vi "4.vi"() -> ()   [LabVIEW 2018]
panel:
  out "W":dbl
  in  "Z":dbl
  in  "Y":dbl
  in  "X":dbl
  # "some debugging tools :\ncontext help \nprobe \nexecution highlight\nsingle stepping \nbreak points \nretian wire value"
  # "this VI is designed to substutute on the equation  \n  w=  (x-y)(x+z-y)(z-x)"
  # "testing values :\n\nx=5   y=7  z=3 --> w=4\n\nx=-4  y=-5  z=8 -->w=108"
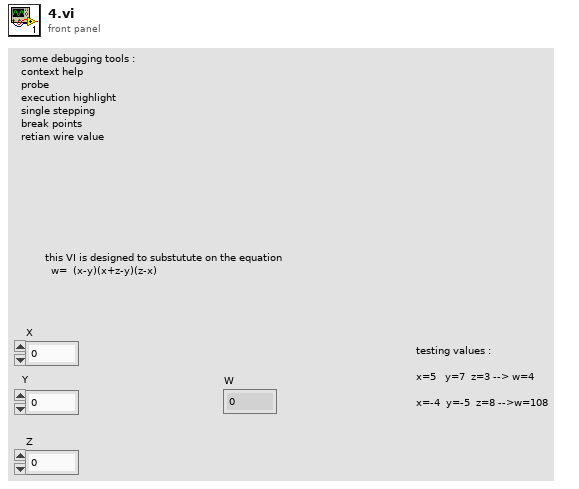
[diagram p1: front panel]
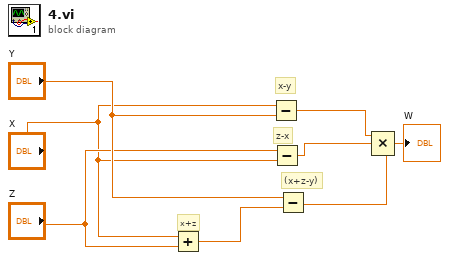
[diagram p0: block diagram]
diagram:
  # "(x+z-y)"
  # "x+z"
  # "z-x"
  # "x-y"
  n1 = Add(x="X", y="Z") -> (x+y=w8:dbl)
  n2 = Subtract(x="X", y="Y") -> (x-y=w4:dbl)
  n3 = Subtract(x="Z", y="X") -> (x-y=w3:dbl)
  n4 = Subtract(x="Y", y=w8) -> (x-y=w2:dbl)
  n5 = Compound Arithmetic op=MULTIPLY(w4, w3, w2) -> (→"W":dbl)
